vi "Reverse2DArray.vi"(11 "In_Arrray":string[][](array[string])) -> (3 "Out_Arrray":string[][](array[string]))   [LabVIEW 2020]
doc: "W LabView nie ma wbudowanej opcji do sortowania tablicy w kolejnoœci od najwiêkszej do najmniejszej. \nVI ten s³u¿y do odwórcenia tablicy posortownej w kolejnoœci od najmniejszej do najwiêkszej."
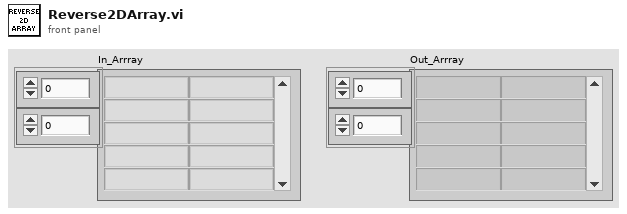
[diagram p1: front panel]
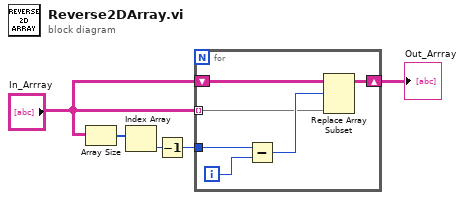
[diagram p0: block diagram]
diagram:
  n1 = Array Size(array="In_Arrray") -> (size(s)=w5:i32[])
  n2 = Index Array(array=w5) -> (element=w4:i32)  [unwired: 1 in]
  n3 = Decrement(x=w4) -> (x-1=w3:i32)
  n4 = for {
    tunnel: "In_Arrray" -> [w8] mode=indexing
    tunnel: w3 -> [w11]
    shift-right: [w6] -> w1
    shift-left: "In_Arrray" -> [w10]
    i -> [w7]
    n5 = Subtract(x=w11, y=w7) -> (x-y=w9:i32)
    n6 = Replace Array Subset(array=w10, new element=w8, index (row)=w9) -> (w6:string[][])  [unwired: 1 in]
  }
  "Out_Arrray" <- w1
